vi "JSON to LVObject.vi"(7 "Theme Serializer in":refnum<class "Theme Serializer.lvclass">, 8 "error in":errorcluster, 9 "Object Type":refnum<class>, 10 "Offset":i32, 11 "JSON":string) -> (0 "error out":errorcluster, 1 "Object":refnum<class>)   [LabVIEW 2021, in "Theme Serializer.lvclass"]
doc: "Convert JSON to an Object of a LabVIEW Class.\n\n<b>Code Developed By:</b> +\nDaniel Coons +\nTechnology Service Corporation +\nwww.tsc.com/atcs"
uses:
  Theme Serializer.lvclass
  Theme Config/Theme Config.lvclass
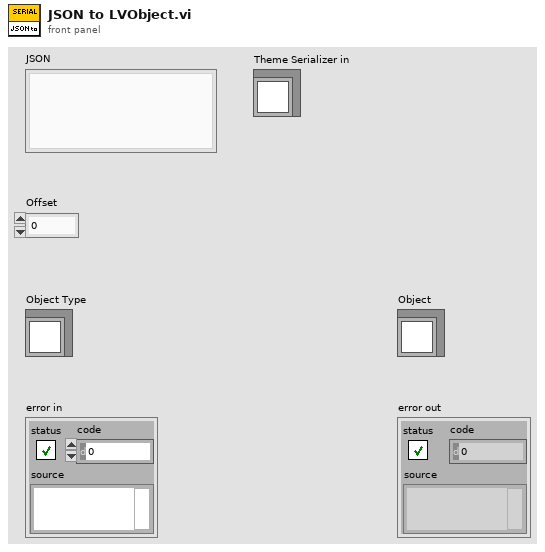
[diagram p1: front panel]
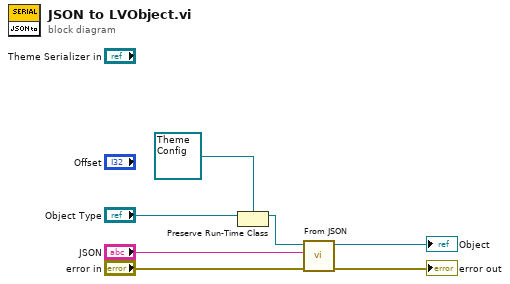
[diagram p0: block diagram]
diagram:
  n1 = Preserve Run-Time Class(object in="Object Type", 2:refnum<class "Theme Config.lvclass"> refnum ("Theme Config.lvclass")) -> (object out=w3:refnum<class "Theme Config.lvclass">)  [unwired: 1 in, 1 out]
  n2 = call "From JSON.vi"("error in"="error in", "JSON"="JSON", "Theme Config in"=w3) -> ("error out"=→"error out":errorcluster, "Theme Config out"=→"Object":refnum<class "Theme Config.lvclass">)  [unwired: 7 in]
